vi "Sweep.vi"(0 "SPU":refnum<k24>, 1 "Refdata_struct":refnum<k24>[](array[refnum]), 2 "TSL":refnum<k24>, 3 "Ref_monitordata_struct":refnum<k24>[](array[refnum]), 4 "ILSTS":refnum<k24>, 5 "错误输入（无错误）":errorcluster, 10 "MPM":refnum<k24>[](array[refnum]), 12 "chkeach_ch":bool) -> (19 "错误输出":errorcluster)   [LabVIEW 2017]
doc: "Get Reference"
uses:
  D:/test/ILSTS/LV_IL_Sample/DLL/STSProcess.dll
  DLL/STSProcess.dll
  D:/test/ILSTS/LV_IL_Sample/DLL/InstrumentDLL.dll
  DLL/InstrumentDLL.dll
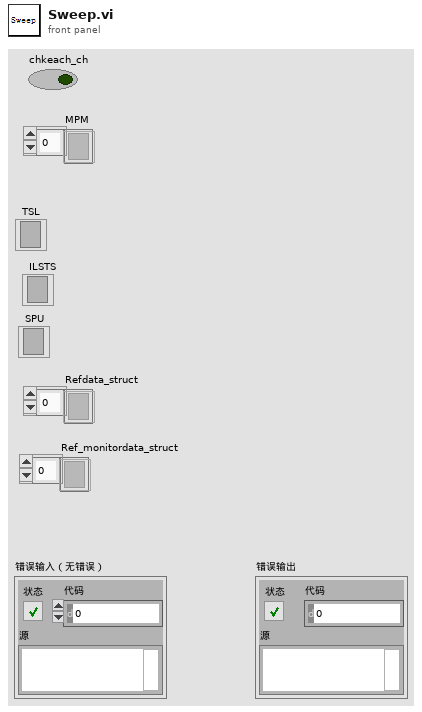
[diagram p1: front panel]
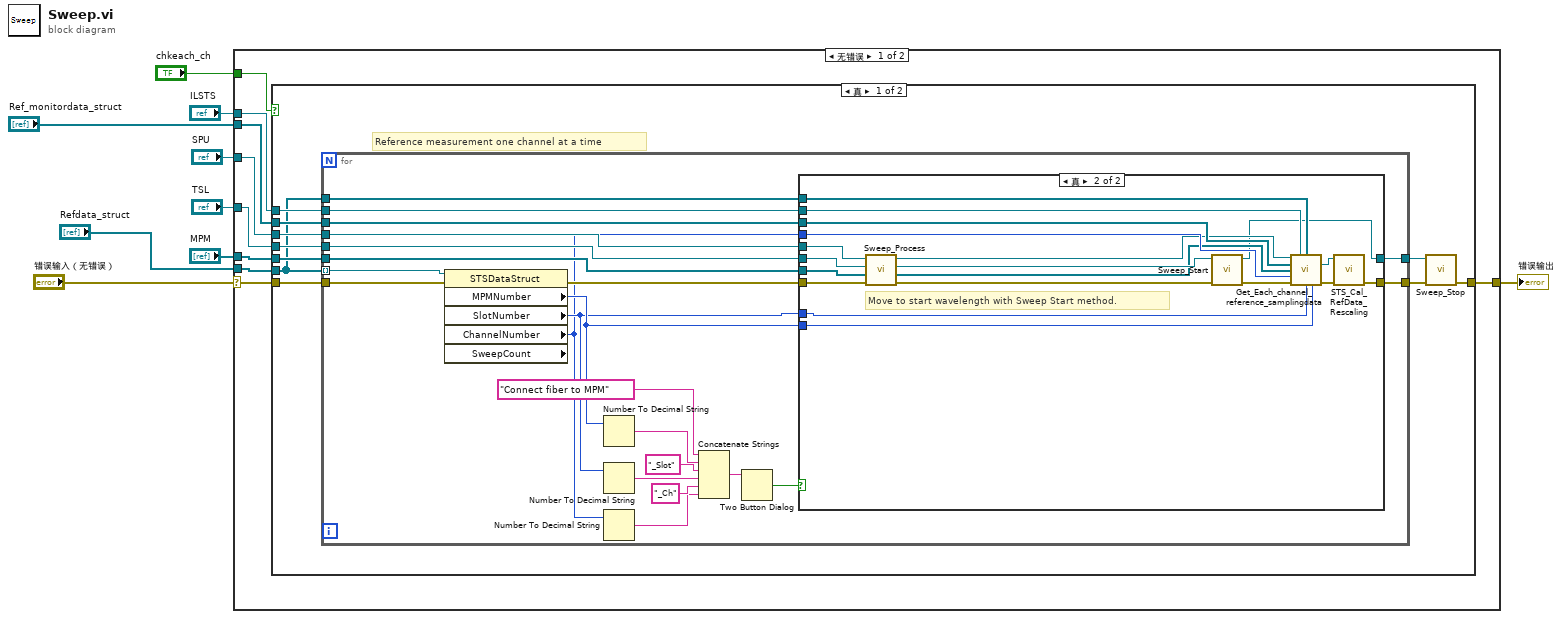
[diagram p0: block diagram]
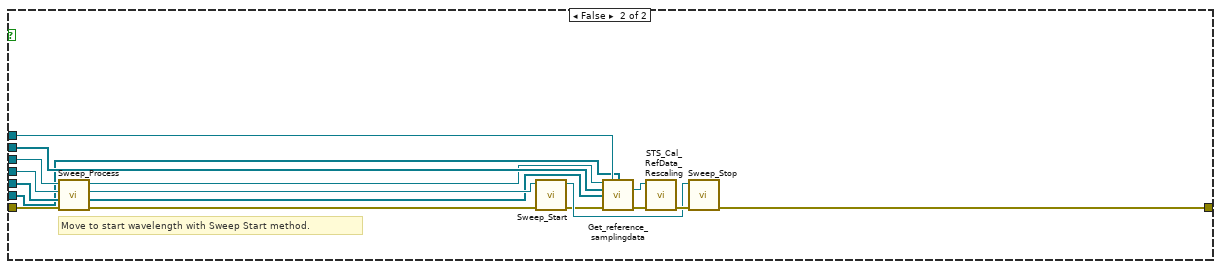
[diagram p3: hidden frame]
diagram:
  n1 = case shown="无错误" "错误输入（无错误）" {
    selector: "错误输入（无错误）" -> [w10 w89]
    tunnel: "Ref_monitordata_struct" -> [w18 _]
    tunnel: "ILSTS" -> [w17 _]
    tunnel: [w16 w89] -> w8
    tunnel: "SPU" -> [w15 _]
    tunnel: "MPM" -> [w14 _]
    tunnel: "TSL" -> [w13 _]
    tunnel: "chkeach_ch" -> [w12 _]
    tunnel: "Refdata_struct" -> [w11 _]
    frame No Error {
      n2 = case shown="真" w12 {
        tunnel: w13 -> [w26 w86]
        tunnel: w14 -> [w28 w88]
        tunnel: w15 -> [w27 w87]
        tunnel: w10 -> [w25 w85]
        tunnel: [w19 w84] -> w16
        tunnel: w11 -> [w22 w81]
        tunnel: w17 -> [w24 w83]
        tunnel: w18 -> [w23 w82]
        frame True {
          # "Reference measurement one channel at a time"
          n3 = for {
            tunnel: w26 -> [w42]
            tunnel: w28 -> [w40]
            tunnel: w27 -> [w41]
            tunnel: w25 -> [w35]
            tunnel: w22 -> [w34] mode=indexing
            tunnel: w24 -> [w33]
            tunnel: w22 -> [w32]
            tunnel: w23 -> [w31]
            tunnel: [w29] -> w21
            tunnel: [w30] -> w20
            n4 = property on="属性节点" class="STSDataStruct" props=["MPMNumber", "SlotNumber", "ChannelNumber", "SweepCount"](reference=w34, error in=w35) -> (error out=w43:errorcluster, "MPMNumber"=w39:i32, "SlotNumber"=w38:i32, "ChannelNumber"=w37:i32)  [unwired: 2 out]
            n5 = Number To Decimal String(number=w39) -> (decimal integer string=w49:string)  [unwired: 1 in]
            n6 = Number To Decimal String(number=w38) -> (decimal integer string=w47:string)  [unwired: 1 in]
            n7 = Number To Decimal String(number=w37) -> (decimal integer string=w45:string)  [unwired: 1 in]
            n8 = Concatenate Strings("Connect fiber to MPM" ("消息"), w49, "_Slot" ("字符串"), w47, "_Ch" ("字符串"), w45) -> (w44:string)
            n9 = Two Button Dialog(message=w44) -> (T button?=w36:bool)  [unwired: 2 in]
            n10 = case shown="真" w36 {
              tunnel: w43 -> [w52 w71]
              tunnel: w42 -> [w51 w70]
              tunnel: w41 -> [_ w69]
              tunnel: w40 -> [_ w68]
              tunnel: w39 -> [_ w67]
              tunnel: w38 -> [_ w66]
              tunnel: w37 -> [_ w65]
              tunnel: w33 -> [_ w64]
              tunnel: [w52 w53] -> w29
              tunnel: w32 -> [_ w63]
              tunnel: w31 -> [_ w62]
              tunnel: [w51 w54] -> w30
              frame False {
              }
              frame True {
                # "Move to start wavelength with Sweep Start method."
                n11 = call "Sweep_Process.vi"("错误输入（无错误）"=w71, "MPM"=w68, "TSL"=w70, "SPU"=w69) -> ("error out"=w61:errorcluster, "MPM out"=w57:refnum<k24>[], "TSL out"=w58:refnum<k24>, "SPU out"=w56:refnum<k24>)  [unwired: 4 in]
                n12 = call "Sweep_Start.vi"("error in (no error)"=w61, ".NET Reference in"=w58) -> ("error out"=w60:errorcluster, "Reference out"=w54:refnum<k24>)  [unwired: 8 in]
                n13 = call "Get_Each_channel_reference_samplingdata.vi"("SPU"=w56, "STSProcess.ILSTS"=w64, "Refdata_struct"=w63, "Ref_monitordata_struct"=w62, "MPM"=w57, "ChannelNumber"=w65, "错误输入（无错误）"=w60, "SlotNumber"=w66, "MPMNumber"=w67) -> ("ILSTS out"=w55:refnum<k24>, "error out"=w59:errorcluster)  [unwired: 5 in]
                n14 = call "STS_Cal_RefData_Rescaling.vi"("错误输入（无错误）"=w59, "ILSTS"=w55) -> ("error out"=w53:errorcluster)  [unwired: 8 in, 1 out]
              }
            }
          }
          n15 = call "Sweep_Stop.vi"("error in (no error)"=w21, ".NET Reference in"=w20) -> ("error out"=w19:errorcluster)  [unwired: 8 in, 1 out]
        }
        frame False {
          # "Move to start wavelength with Sweep Start method."
          n16 = call "Sweep_Process.vi"("错误输入（无错误）"=w85, "MPM"=w88, "TSL"=w86, "SPU"=w87) -> ("error out"=w80:errorcluster, "MPM out"=w74:refnum<k24>[], "TSL out"=w75:refnum<k24>, "SPU out"=w73:refnum<k24>)  [unwired: 4 in]
          n17 = call "Sweep_Start.vi"("error in (no error)"=w80, ".NET Reference in"=w75) -> ("error out"=w77:errorcluster, "Reference out"=w78:refnum<k24>)  [unwired: 8 in]
          n18 = call "Get_reference_samplingdata.vi"("SPU"=w73, "STSProcess.ILSTS"=w83, "Refdata_struct"=w81, "Ref_monitordata_struct"=w82, "MPM"=w74, "错误输入（无错误）"=w77) -> ("ILSTS out"=w72:refnum<k24>, "error out"=w76:errorcluster)  [unwired: 8 in]
          n19 = call "STS_Cal_RefData_Rescaling.vi"("错误输入（无错误）"=w76, "ILSTS"=w72) -> ("error out"=w79:errorcluster)  [unwired: 8 in, 1 out]
          n20 = call "Sweep_Stop.vi"("error in (no error)"=w79, ".NET Reference in"=w78) -> ("error out"=w84:errorcluster)  [unwired: 8 in, 1 out]
        }
      }
    }
    frame Error {
    }
  }
  "错误输出" <- w8
